vi "Initialize.vi"(7 "Process ID":string, 8 "error in (no error)":errorcluster, 10 "Device Item Ref":T1=18446744073709551615 format="%.0x", 11 "Assembler in":refnum<class "Assembler.lvclass">) -> (0 "error out":errorcluster, 3 "Assembler out":refnum<class "Assembler.lvclass">)   [LabVIEW 2019, in "TimingDRV Engine.lvlib" / "Assembler.lvclass"]
uses:
  Assembler.lvclass
  C:/Users/XEnderMD/Desktop/CD Project Tools/Source/Engine/Windows/Parent Classes/Process/Process.lvclass
  <vilib>/NI VeriStand/Custom Device API/Custom Device Item Ref.ctl
  Assembler.lvclass/Assembler.ctl
  Parent Classes/Process/Process.lvclass/Process.ctl
  Parent Classes/Process/Accessors/Process ID/Get Process ID.vi
  Parent Classes/Process/Accessors/Process UEs/Set Process UEs.vi
  Parent Classes/Process/Accessors/Process Qs/Set Process Qs.vi
  Parent Classes/Process/Accessors/Process IDs/Set Process IDs.vi
  Parent Classes/Process/Process.lvclass
  <vilib>/NI VeriStand/Custom Device API/Custom Device API.lvlib
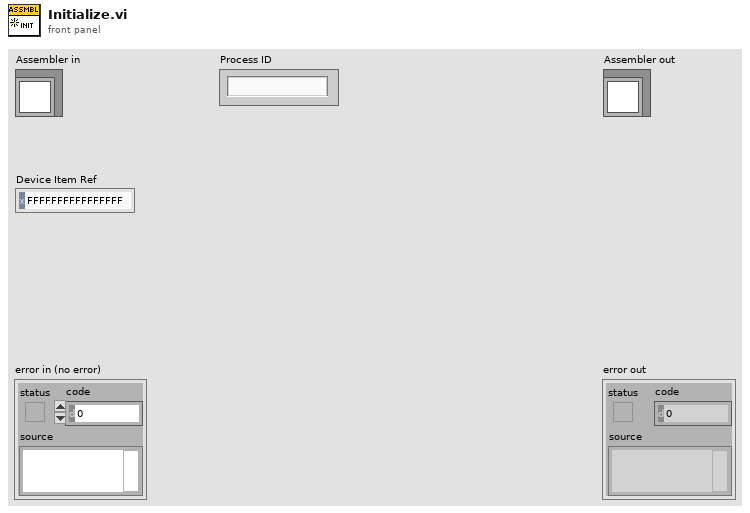
[diagram p1: front panel]
types:
  T1 = typedef "Custom Device API.lvlib/Custom Device Item Ref.ctl" = u64
  T2 = typedef "TimingDRV Engine.lvlib/Process.lvclass/Process Lookup.ctl" = cluster{"Process ID":string, "MessageQ":refnum<queue>, "Update UE":refnum<user-event>}
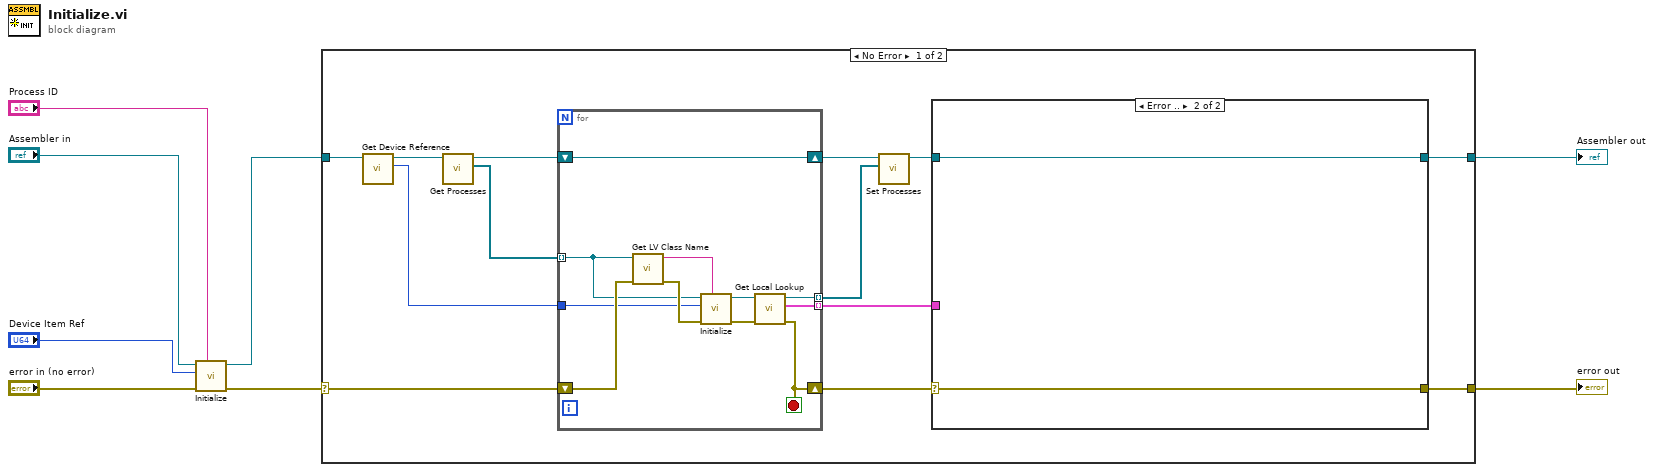
[diagram p0: block diagram]
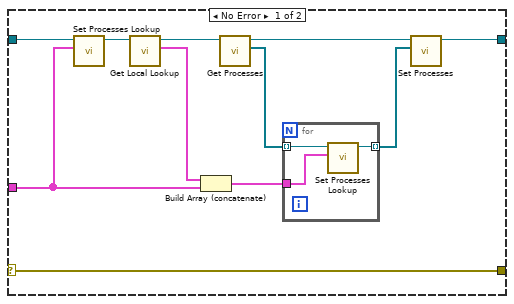
[diagram p2: hidden frame]
diagram:
  n1 = call-parent "Initialize.vi"("Process ID"="Process ID", "error in (no error)"="error in (no error)", "Device Item Ref"="Device Item Ref", "Process in"="Assembler in") -> ("error out"=w2:errorcluster, "Process out"=w3:refnum<class "Assembler.lvclass">)  [unwired: 6 in]
  n2 = case shown="No Error" w2 {
    selector: w2 -> [w21 w49]
    tunnel: w3 -> [w10 w50]
    tunnel: [w14 w50] -> w4
    tunnel: [w13 w49] -> w1
    frame No Error {
      n3 = call "Get Device Reference.vi"("CD_Process in"=w10) -> ("Device Item Ref"=w20:T1, "CD_Process out"=w11:refnum<class "Assembler.lvclass">)  [unwired: 9 in]
      n4 = call "Get Processes.vi"("Assembler in"=w11) -> ("Processes"=w12:refnum<class "Process.lvclass">[], "Assembler out"=w9:refnum<class "Assembler.lvclass">)  [unwired: 9 in]
      n5 = for {
        tunnel: w12 -> [w45] mode=indexing
        shift-right: [w43] -> w19
        shift-left: w9 -> [w43]
        tunnel: w20 -> [w44]
        shift-right: [w39] -> w16
        shift-left: w21 -> [w46]
        tunnel: [w41] -> w18 mode=indexing
        tunnel: [w38] -> w15 mode=indexing
        stop <- w39 stop-if-true
        n6 = call <vilib>:"Get LV Class Name.vi"("error in (no error)"=w46, "object"=w45) -> ("error out"=w48:errorcluster, "class name"=w47:string)  [unwired: 8 in]
        n7 = call-dynamic "Initialize.vi"("Process ID"=w47, "error in (no error)"=w48, "Device Item Ref"=w44, "Process in"=w45) -> ("error out"=w40:errorcluster, "Process out"=w42:refnum<class "Process.lvclass">)  [unwired: 6 in]
        n8 = call-dynamic "Get Local Lookup.vi"("error in (no error)"=w40, "Process in"=w42) -> ("error out"=w39:errorcluster, "Process Lookup"=w38:T2, "Process out"=w41:refnum<class "Process.lvclass">)  [unwired: 7 in]
      }
      n9 = call "Set Processes.vi"("Processes"=w18, "Assembler in"=w19) -> ("Assembler out"=w17:refnum<class "Assembler.lvclass">)  [unwired: 9 in]
      n10 = case shown="Error .." w16 {
        selector: w16 -> [w25 w36]
        tunnel: w17 -> [w24 w37]
        tunnel: w15 -> [w22 _]
        tunnel: [w26 w37] -> w14
        tunnel: [w25 w36] -> w13
        frame No Error {
          n11 = call "Set Processes Lookup.vi"("Processes Lookup"=w22, "Process in"=w24) -> ("Process out"=w23:refnum<class "Assembler.lvclass">)  [unwired: 9 in]
          n12 = call-dynamic "Get Local Lookup.vi"("Process in"=w23) -> ("Process Lookup"=w29:T2, "Process out"=w30:refnum<class "Assembler.lvclass">)  [unwired: 8 in, 1 out]
          n13 = Build Array (concatenate)(w29, w22) -> (w28:T2[])
          n14 = call "Get Processes.vi"("Assembler in"=w30) -> ("Processes"=w32:refnum<class "Process.lvclass">[], "Assembler out"=w31:refnum<class "Assembler.lvclass">)  [unwired: 9 in]
          n15 = for {
            tunnel: w32 -> [w35] mode=indexing
            tunnel: w28 -> [w34]
            tunnel: [w33] -> w27 mode=indexing
            n16 = call "Set Processes Lookup.vi"("Processes Lookup"=w34, "Process in"=w35) -> ("Process out"=w33:refnum<class "Process.lvclass">)  [unwired: 9 in]
          }
          n17 = call "Set Processes.vi"("Processes"=w27, "Assembler in"=w31) -> ("Assembler out"=w26:refnum<class "Assembler.lvclass">)  [unwired: 9 in]
        }
        frame Error {
        }
      }
    }
    frame Error {
    }
  }
  "error out" <- w1
  "Assembler out" <- w4
